vi "Error Query.vi"(8 "error in (no error)":errorcluster, 11 "VISA resource name":refnum<visa-resource-name>) -> (0 "error out":errorcluster, 1 "Error Message":string, 2 "Error Code":i32[](array[numeric]), 3 "VISA resource name out":refnum<visa-resource-name>)   [LabVIEW 2010, in "Agilent 3458.lvlib"]
doc: "Queries the instrument for any errors in the instrument's error queue. It will continue to read errors until all errors have been read from the instrument. Any errors will be returned in the Error Out cluster.\n\nNote:\nThis VI is called automatically by most driver VIs so it is not usually necessary to call this in an application."
uses:
  <instrlib>/Agilent 3458/Agilent 3458.lvlib
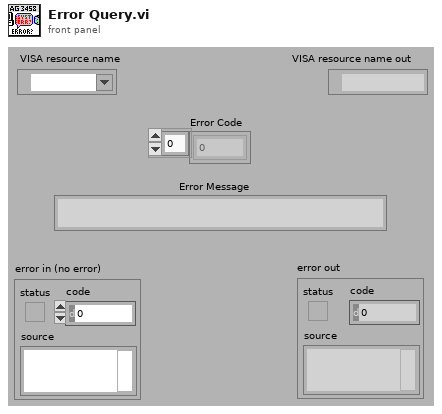
[diagram p1: front panel]
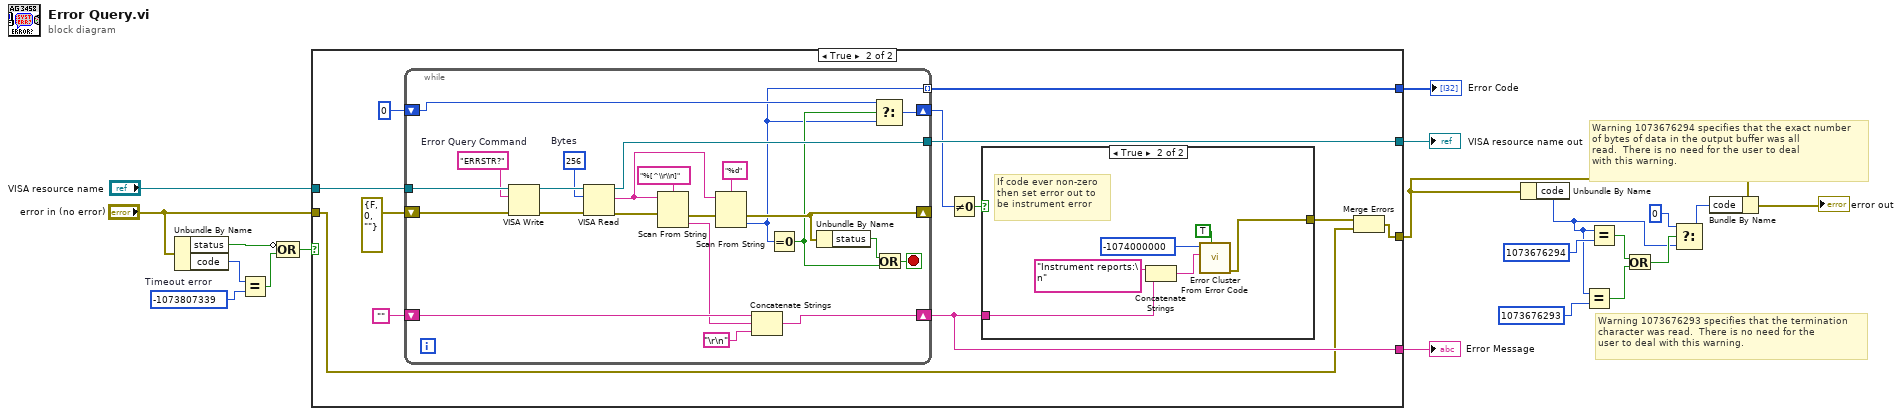
[diagram p0: block diagram]
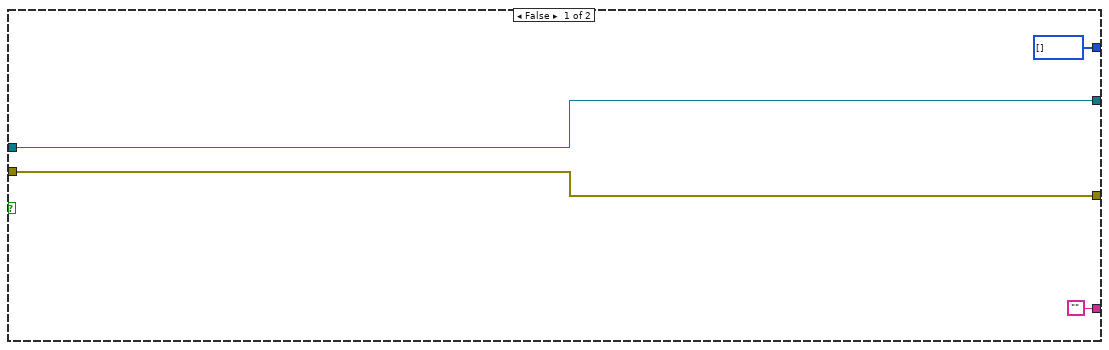
[diagram p2: hidden frame]
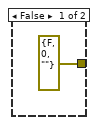
[diagram p3: hidden frame]
diagram:
  w17 = -1073807339  # Timeout error
  # "Warning 1073676293 specifies that the termination \ncharacter was read.  There is no need for the \nuser to deal with this warning."
  # "Warning 1073676294 specifies that the exact number\nof bytes of data in the output buffer was all\nread.  There is no need for the user to deal\nwith this warning."
  n1 = Unbundle By Name("error in (no error)") -> ("status"=w18:bool, "code"=w15:i32)
  n2 = Equal?(x=w15, y=w17) -> (x = y?=w16:bool)
  n3 = Compound Arithmetic op=OR(invert w18, w16) -> (w14:bool)
  n4 = case shown="True" w14 {
    tunnel: [w24 w36] -> w20
    tunnel: "VISA resource name" -> [w24 w35]
    tunnel: "error in (no error)" -> [w23 w25]
    tunnel: [w23 w33] -> w3
    tunnel: ["" w27] -> w13
    tunnel: [i32[] [] w26] -> w12
    frame False {
    }
    frame True {
      n5 = while {
        tunnel: [w66] -> w36
        tunnel: w35 -> [w65]
        shift-right: [w53] -> w27
        shift-left: "" -> [w56]
        shift-right: [w51] -> w28
        shift-left: 0 -> [w52]
        shift-right: [w49] -> _
        shift-left: errorcluster {"status"=FALSE, "code"=0, "source"=""} ("error in (no error)") -> [w50]
        tunnel: [w44] -> w26 mode=indexing
        stop <- w59 stop-if-true
        w63 = u32 256  # Bytes
        w61 = "ERRSTR?"  # Error Query Command
        n6 = VISA Write(VISA resource name=w65, write buffer=w61, error in (no error)=w50) -> (VISA resource name out=w64:refnum<visa-resource-name>, error out=w62:errorcluster)  [unwired: 1 out]
        n7 = VISA Read(VISA resource name=w64, byte count=w63, error in (no error)=w62) -> (VISA resource name out=w66:refnum<visa-resource-name>, read buffer=w57:string, error out=w48:errorcluster)  [unwired: 1 out]
        n8 = Scan From String(format string="%[^\\r\\n]", input string=w57, error in=w48) -> (error out=w47:errorcluster, output 1=w54:string)  [unwired: 2 in, 2 out]
        n9 = Scan From String(format string="%d", input string=w57, error in=w47) -> (error out=w49:errorcluster, output 1=w44:i32)  [unwired: 2 in, 2 out]
        n10 = Concatenate Strings(w56, w54, "\r\n") -> (w53:string)
        n11 = Equal To 0?(x=w44) -> (x = 0?=w45:bool)
        n12 = Unbundle By Name(w49) -> ("status"=w46:bool)
        n13 = Select(t=w52, s=w45, f=w44) -> (s? t:f=w51:i32)
        n14 = Or(x=w46, y=w45) -> (x .or. y?=w59:bool)
      }
      n15 = Not Equal To 0?(x=w28) -> (x != 0?=w31:bool)
      n16 = case shown="True" w31 {
        tunnel: w27 -> [_ w42]
        tunnel: [errorcluster {"status"=FALSE, "code"=0, "source"=""} ("error out") w38] -> w30
        frame False {
        }
        frame True {
          # "If code ever non-zero\nthen set error out to\nbe instrument error"
          n17 = Concatenate Strings("Instrument reports:\n" ("Source"), w42) -> (w39:string)
          n18 = call <vilib>:"Error Cluster From Error Code.vi"("show call chain? (False)"=TRUE, "error message (\"\")"=w39, "error code (0)"=-1074000000 ("Code")) -> ("error out"=w38:errorcluster)  [unwired: 6 in]
        }
      }
      n19 = Merge Errors(w30, w25) -> (w33:errorcluster)
    }
  }
  "VISA resource name out" <- w20
  "Error Message" <- w13
  "Error Code" <- w12
  n20 = Unbundle By Name(w3) -> ("code"=w4:i32)
  n21 = Equal?(x=w4, y=1073676293) -> (x = y?=w7:bool)
  n22 = Equal?(x=w4, y=1073676294) -> (x = y?=w6:bool)
  n23 = Or(x=w6, y=w7) -> (x .or. y?=w5:bool)
  n24 = Select(t=0, s=w5, f=w4) -> (s? t:f=w9:i32)
  n25 = Bundle By Name(cluster=w3, "code"=w9) -> (→"error out":errorcluster)
